vi "update.file.vi"(8 "error in (no error)":errorcluster, 11 "ComicVine_manager in":refnum<class "CV_downloader.lvclass">) -> (0 "error out":errorcluster, 3 "ComicVine_manager out":refnum<class "CV_downloader.lvclass">)   [LabVIEW 2024, in "CV_downloader.lvclass"]
uses:
  CV_downloader.lvclass
  CV_downloader.lvclass/CV_downloader.ctl
  <userlib>/_OpenG.lib/file/file.llb/Strip Path Extension - String__ogtk.vi
  CV_RESTful_Library/CV_RESTful_Lib.lvlib
  CV_Shared_Library/CV_Shared_Library.lvlib
  <vilib>/addons/_JKI.lib/Serialization/JSON/JKI JSON Serialization.lvlib
  <userlib>/_OpenG.lib/file/file.llb/openg_file.lvlib
  comic_manager/manager_daemon/manager_daemon.lvclass
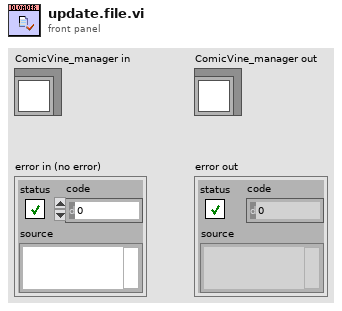
[diagram p1: front panel]
types:
  T1 = typedef "CV_Shared_Library.lvlib/volume.type--enum.ctl" = enum16{"Ongoing", "Limited Series", "Annual", "One Shot", "Reprint/Document", "Star Comics", "Epic Comics"}
  T2 = typedef "CV_RESTful_Lib.lvlib/local_volume--cluster.ctl" = cluster{"id":i32, "name":string, "sortable_name":string, "aliases":string[], "description":string, "site_detail_url":string, "count_of_issues":i32, "start_year":i32, "publisher_id":i32, "issue_ids":i32[], "date_last_updated":timestamp, "volume":i32, "cv_id":string, "volume type":T1}
  T3 = typedef "CV_RESTful_Lib.lvlib/local_issue--cluster.ctl" = cluster{"cover_date":timestamp, "id":i32, "cv_id":string, "name":string, "sortable_name":string, "issue_number":string, "deck":string, "description":string, "volume":T4, "store_date":timestamp, "date_last_updated":timestamp, "site_detail_url":string, "cover_url":string, "associated_images":T5[], "characters":T4[], "concepts":T4[], "creators":T6[], "storyArcs":T4[], "teams":T4[]}
  T4 = typedef "CV_RESTful_Lib.lvlib/cv_issue.generic_credit--cluster.ctl" = cluster{"id":i32, "name":string}
  T5 = typedef "CV_RESTful_Lib.lvlib/cv_issue.associated_image--cluster.ctl" = cluster{"original_url":string, "id":i32}
  T6 = typedef "CV_RESTful_Lib.lvlib/cv_issue.person_credit--cluster.ctl" = cluster{"id":i32, "name":string, "role":string}
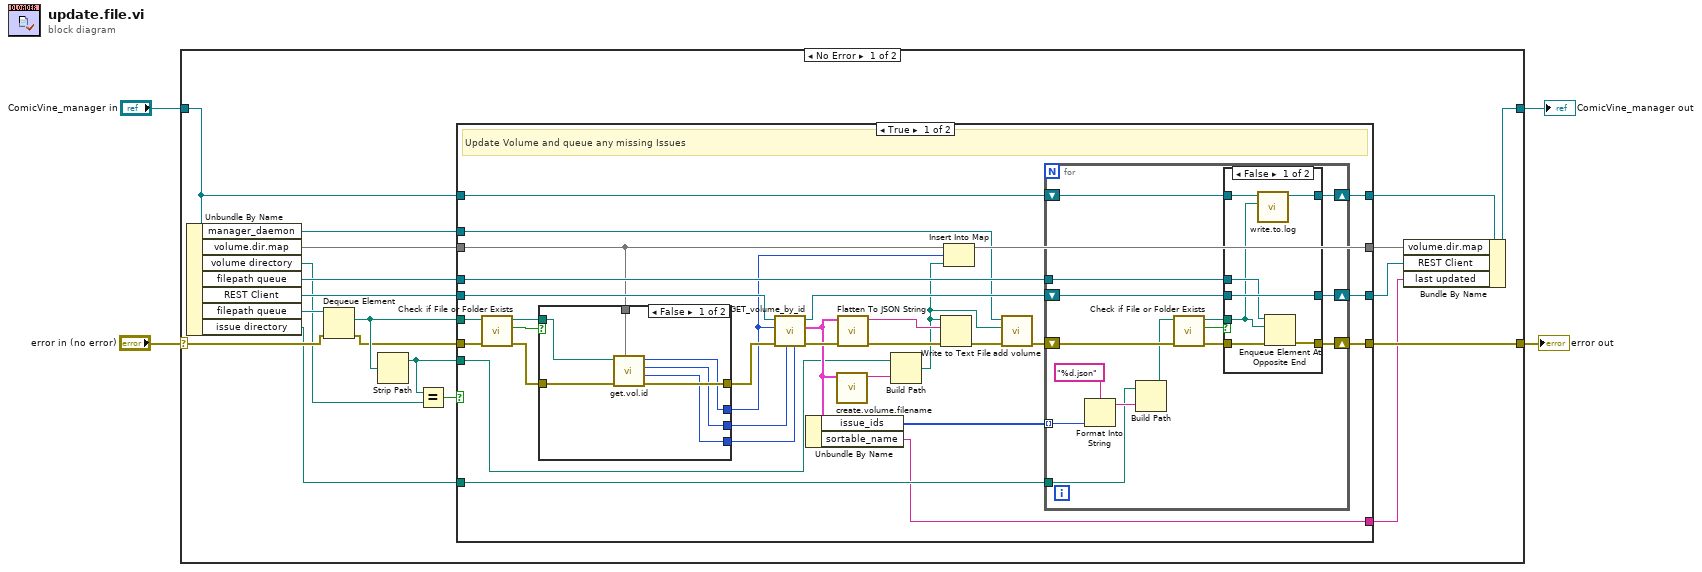
[diagram p0: block diagram]
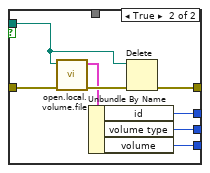
[diagram p2: hidden frame]
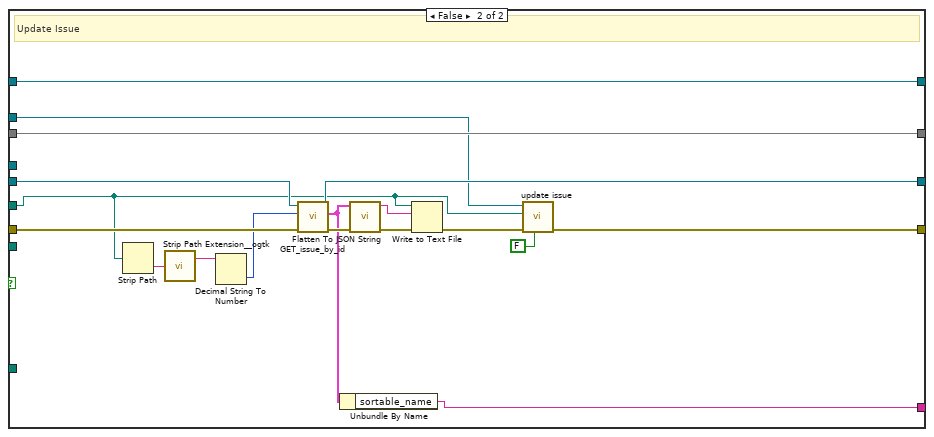
[diagram p4: hidden frame]
diagram:
  n1 = case shown="No Error" "error in (no error)" {
    selector: "error in (no error)" -> [w22 w114]
    tunnel: [w19 w114] -> w3
    tunnel: [w17 w113] -> w1
    tunnel: "ComicVine_manager in" -> [w8 w113]
    frame No Error {
      n2 = Unbundle By Name(w8) -> ("manager_daemon"=w6:refnum<class "manager_daemon.lvclass">, "volume.dir.map"=w11:map{i32, path}, "volume directory"=w15:path, "filepath queue"=w16:refnum<queue>, "REST Client"=w21:refnum<class "REST Client.lvclass">, "filepath queue"=w23:refnum<queue>, "issue directory"=w9:path)
      n3 = Dequeue Element(queue=w23, error in (no error)=w22) -> (element=w20:path, error out=w12:errorcluster)  [unwired: 1 in, 2 out]
      n4 = Strip Path(path=w20) -> (stripped path=w14:path)  [unwired: 1 out]
      n5 = Equal?(x=w14, y=w15) -> (x = y?=w13:bool)
      n6 = case shown="True" w13 {
        tunnel: w21 -> [w54 w112]
        tunnel: w12 -> [w43 w111]
        tunnel: w20 -> [w42 w98]
        tunnel: w14 -> [w41 _]
        tunnel: [w45 w100] -> w19
        tunnel: [w47 w107] -> w18
        tunnel: w16 -> [w44 _]
        tunnel: w11 -> [w35 w106]
        tunnel: [w33 w106] -> w10
        tunnel: w9 -> [w32 _]
        tunnel: w8 -> [w31 w102]
        tunnel: [w30 w102] -> w7
        tunnel: w6 -> [w24 w99]
        tunnel: [w28 w95] -> w5
        frame True {
          # "Update Volume and queue any missing Issues"
          n7 = call <vilib>:"Check if File or Folder Exists.vi"("error in (no error)"=w43, "path"=w42) -> ("error out"=w37:errorcluster, "file or folder exists?"=w38:bool, "dup path"=w40:path)  [unwired: 7 in]
          n8 = case shown="False" w38 {
            tunnel: [w56 w67] -> w34
            tunnel: w40 -> [w58 w66]
            tunnel: [w57 w65] -> w39
            tunnel: w37 -> [w60 w64]
            tunnel: [w61 w63] -> w36
            tunnel: w35 -> [w59 _]
            tunnel: [w55 w62] -> w29
            frame False {
              n9 = call "get.vol.id.vi"("map in"=w59, "error in (no error)"=w60, "Path"=w58) -> ("error out"=w61:errorcluster, "volume"=w55:i32, "volume type"=w57:T1, "id"=w56:i32)  [unwired: 5 in]
            }
            frame True {
              n10 = call "open.local.volume.file.vi"("error in (no error)"=w64, "volume json"=w66) -> ("error out"=w69:errorcluster, "volume"=w68:T2)  [unwired: 8 in]
              n11 = Unbundle By Name(w68) -> ("id"=w67:i32, "volume type"=w65:T1, "volume"=w62:i32)
              n12 = Delete(path (use dialog)=w66, error in=w69) -> (error out=w63:errorcluster)  [unwired: 3 in, 2 out]
            }
          }
          n13 = call "GET_volume_by_id.vi"("volume"=w29, "volume type"=w39, "error in (no error)"=w36, "volume id"=w34, "REST Client in"=w54) -> ("error out"=w52:errorcluster, "local volume"=w49:T2, "REST Client out"=w48:refnum<class "REST Client.lvclass">)  [unwired: 4 in]
          n14 = Unbundle By Name(w49) -> ("issue_ids"=w46:i32[], "sortable_name"=w28:string)
          n15 = call "create.volume.filename.vi"("volume"=w49) -> ("json filename"=w53:string)  [unwired: 10 in]
          n16 = call <vilib>:"Flatten To JSON String.vi"("error in"=w52, "Variant"=w49) -> ("error out"=w50:errorcluster, "JSON String"=w51:string)  [unwired: 8 in]
          n17 = Build Path(base path=w41, name or relative path=w53) -> (appended path=w25:path)
          n18 = Write to Text File(file (use dialog)=w25, text=w51, error in=w50) -> (error out=w27:errorcluster)  [unwired: 1 in, 2 out]
          n19 = Insert Into Map(map in=w35, key=w34, value=w25) -> (map out=w33:map{i32, path})  [unwired: 2 out]
          n20 = call "add volume.vi"("error in (no error)"=w27, "Volume Path"=w25, "manager_daemon in"=w24) -> ("error out"=w26:errorcluster)  [unwired: 7 in, 1 out]
          n21 = for {
            shift-right: [w74] -> w47
            shift-left: w48 -> [w75]
            tunnel: w46 -> [w83] mode=indexing
            tunnel: w32 -> [w81]
            shift-right: [w76] -> w45
            shift-left: w26 -> [w80]
            tunnel: w44 -> [w73]
            shift-right: [w70] -> w30
            shift-left: w31 -> [w71]
            n22 = Format Into String(format string="%d.json", w83) -> (resulting string=w82:string)  [unwired: 2 in, 1 out]
            n23 = Build Path(base path=w81, name or relative path=w82) -> (appended path=w79:path)
            n24 = call <vilib>:"Check if File or Folder Exists.vi"("error in (no error)"=w80, "path"=w79) -> ("error out"=w77:errorcluster, "file or folder exists?"=w78:bool, "dup path"=w72:path)  [unwired: 7 in]
            n25 = case shown="False" w78 {
              tunnel: w77 -> [w90 w94]
              tunnel: [w88 w94] -> w76
              tunnel: w75 -> [w91 w93]
              tunnel: [w91 w93] -> w74
              tunnel: w73 -> [w89 _]
              tunnel: w72 -> [w86 _]
              tunnel: w71 -> [w87 w92]
              tunnel: [w85 w92] -> w70
              frame False {
                n26 = call "write.to.log"("new path"=w86, "ComicVine_manager in"=w87) -> ("ComicVine_manager out"=w85:refnum<class "CV_downloader.lvclass">)  [unwired: 8 in, 1 out]
                n27 = Enqueue Element At Opposite End(queue=w89, element=w86, error in (no error)=w90) -> (error out=w88:errorcluster)  [unwired: 1 in, 2 out]
              }
              frame True {
              }
            }
          }
        }
        frame False {
          # "Update Issue"
          n28 = Strip Path(path=w98) -> (name=w105:string)  [unwired: 1 out]
          n29 = call-poly <userlib>:"Strip Path Extension__ogtk.vi"("path"=w105) -> ("root"=w104:string)  [unwired: 1 out]
          n30 = Decimal String To Number(string=w104) -> (number=w103:i32)  [unwired: 2 in, 1 out]
          n31 = call "GET_issue_by_id.vi"("error in (no error)"=w111, "issue id"=w103, "REST Client in"=w112) -> ("error out"=w110:errorcluster, "local_issue"=w96:T3, "REST Client out"=w107:refnum<class "REST Client.lvclass">)  [unwired: 6 in]
          n32 = Unbundle By Name(w96) -> ("sortable_name"=w95:string)
          n33 = call <vilib>:"Flatten To JSON String.vi"("error in"=w110, "Variant"=w96) -> ("error out"=w109:errorcluster, "JSON String"=w108:string)  [unwired: 8 in]
          n34 = Write to Text File(file (use dialog)=w98, text=w108, error in=w109) -> (error out=w101:errorcluster)  [unwired: 1 in, 2 out]
          n35 = call "update issue.vi"("Update All (T)"=FALSE, "error in (no error)"=w101, "Issue Path"=w98, "manager_daemon in"=w99) -> ("error out"=w100:errorcluster)  [unwired: 6 in, 1 out]
        }
      }
      n36 = Bundle By Name(cluster=w7, "volume.dir.map"=w10, "REST Client"=w18, "last updated"=w5) -> (w17:refnum<class "CV_downloader.lvclass">)
    }
    frame Error {
    }
  }
  "error out" <- w3
  "ComicVine_manager out" <- w1
